vi "uniform (SubVI).vi"(6 "seed":i32=-1, 7 "reset":bool, 9 "xmax":dbl=1.0, 10 "xmin":dbl, 11 "samples":i32=128) -> ()   [LabVIEW 2011]
panel:
  out "Array":cluster{"x":dbl, "y":dbl}[](array[cluster])
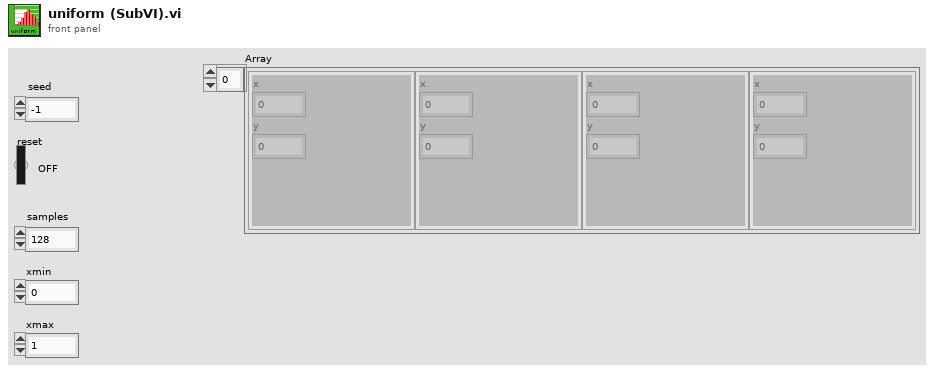
[diagram p1: front panel]
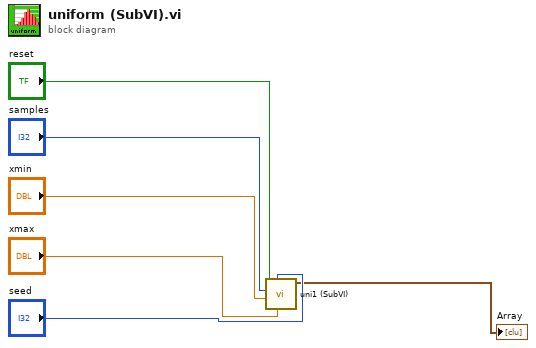
[diagram p0: block diagram]
diagram:
  n1 = call "uni1 (SubVI).vi"("xmax"="xmax", "seed"="seed", "xmin"="xmin", "samples"="samples", "reset"="reset") -> ("Array"=→"Array":cluster{"x":dbl, "y":dbl}[])  [unwired: 6 in]
